vi "find_existing_controls.vi"(8 "error in (no error)":errorcluster, 10 "Label Text":string, 11 "VI Ref In":refnum<vi>) -> (0 "error out":errorcluster, 1 "New Ctrl":bool, 2 "Ctrl Ref Out":refnum<vi>, 3 "VI Ref Out":refnum<vi>)   [LabVIEW 2018]
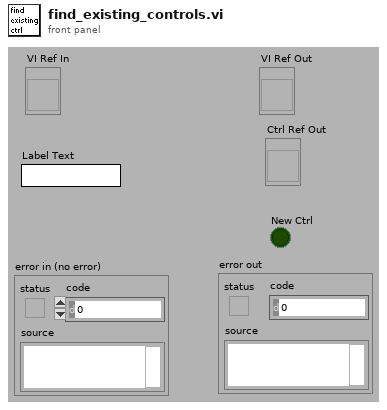
[diagram p1: front panel]
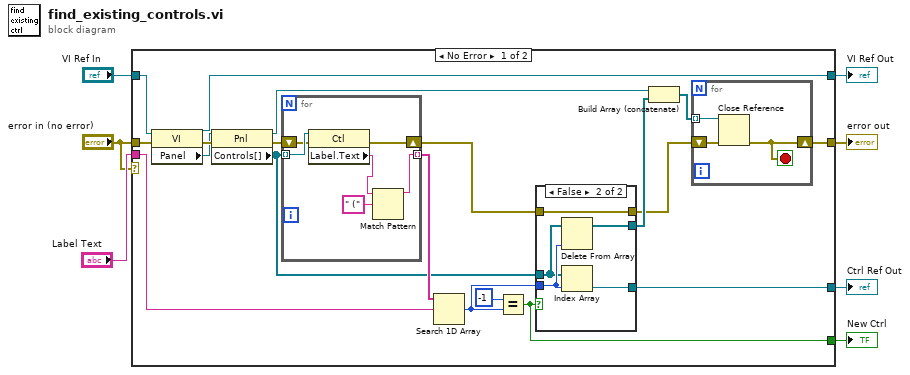
[diagram p0: block diagram]
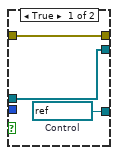
[diagram p2: hidden frame]
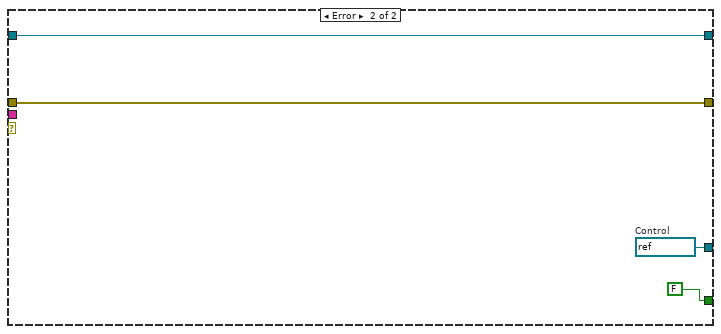
[diagram p3: hidden frame]
diagram:
  n1 = case shown="No Error" "error in (no error)" {
    tunnel: [w21 FALSE] -> w7
    tunnel: [w20 w46] -> w6
    tunnel: "error in (no error)" -> [w19 w47]
    tunnel: [w12 w47] -> w5
    tunnel: "Label Text" -> [w11 _]
    tunnel: "VI Ref In" -> [w10 w44]
    tunnel: [w8 w44] -> w1
    frame No Error {
      n2 = property class="VI"(reference=w10, error in=w19) -> (reference out=w8:refnum<vi>, error out=w25:errorcluster, "Panel"=w18:refnum<vi>)
      n3 = property class="Pnl"(reference=w18, error in=w25) -> (reference out=w17:refnum<vi>, error out=w24:errorcluster, "Controls[]"=w9:refnum<vi>[])
      n4 = for {
        tunnel: w9 -> [w43] mode=indexing
        tunnel: [w38] -> w26 mode=indexing
        shift-right: [w41] -> w16
        shift-left: w24 -> [w42]
        n5 = property class="Ctl"(reference=w43, error in=w42) -> (error out=w41:errorcluster, "Label.Text"=w39:string)  [unwired: 1 out]
        n6 = Match Pattern(string=w39, regular expression=" (") -> (before substring=w38:string)  [unwired: 4 out]
      }
      n7 = Search 1D Array(1D array=w26, element=w11) -> (index of element=w22:i32)  [unwired: 1 out]
      n8 = Equal?(x=-1, y=w22) -> (x = y?=w21:bool)
      n9 = case shown="False" w21 {
        tunnel: w9 -> [w30 w34]
        tunnel: w22 -> [_ w35]
        tunnel: [w32 w37] -> w20
        tunnel: [w31 w36] -> w14
        tunnel: w16 -> [w31 w36]
        tunnel: [w30 w33] -> w15
        frame True {
          w32 = refnum<vi> refnum  # Control
        }
        frame False {
          n10 = Delete From Array(array=w34, index=w35) -> (array with subset deleted=w33:refnum<vi>[])  [unwired: 1 in, 1 out]
          n11 = Index Array(array=w34, index=w35) -> (element=w37:refnum<vi>)
        }
      }
      n12 = Build Array (concatenate)(w17, w15) -> (w13:refnum<vi>[])
      n13 = for {
        shift-right: [w27] -> w12
        shift-left: w14 -> [w29]
        tunnel: w13 -> [w28] mode=indexing
        stop <- w27 stop-if-true
        n14 = Close Reference(reference=w28, error in (no error)=w29) -> (error out=w27:errorcluster)
      }
    }
    frame Error {
      w46 = refnum<vi> refnum  # Control
    }
  }
  "Ctrl Ref Out" <- w6
  "New Ctrl" <- w7
  "error out" <- w5
  "VI Ref Out" <- w1
